vi "testDoubleArrayToStringWithBrackets.vi"(8 "error in (no error)":errorcluster) -> (0 "error out":errorcluster)   [LabVIEW 2018]
uses:
  <vilib>/addons/_JKI Toolkits/Caraya/classes/Assert/Assert Equal Value_Variant.vi
  <vilib>/addons/_JKI Toolkits/Caraya/classes/Test/Test.lvclass
  <vilib>/addons/_JKI Toolkits/Caraya/classes/Assert/Assert.lvclass
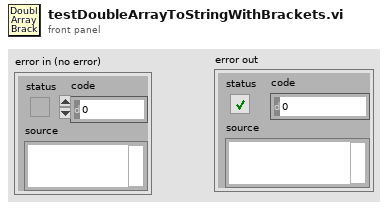
[diagram p1: front panel]
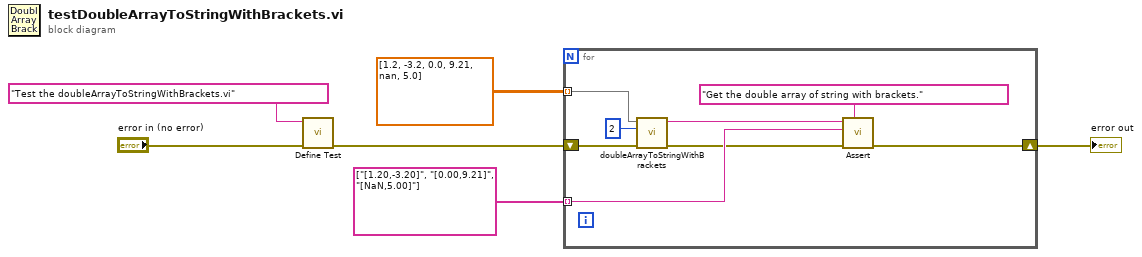
[diagram p0: block diagram]
diagram:
  n1 = call <vilib>:"Define Test.vi"("error in (no error)"="error in (no error)", "Label (VI Title)"="Test the doubleArrayToStringWithBrackets.vi") -> ("error out"=w1:errorcluster)  [unwired: 9 in]
  n2 = for {
    tunnel: string[] ["[1.20,-3.20]", "[0.00,9.21]", "[NaN,5.00]"] ("name") -> [w13] mode=indexing
    shift-right: [w12] -> w3
    shift-left: w1 -> [w8]
    tunnel: dbl[][] [[1.2, -3.2], [0.0, 9.21], [nan, 5.0]] ("value") -> [w11] mode=indexing
    n3 = call "doubleArrayToStringWithBrackets.vi"("error in (no error)"=w8, "presicion (0)"=u8 2, "value"=w11) -> ("error out"=w7:errorcluster, "String"=w10:string)  [unwired: 7 in]
    n4 = call-poly <vilib>:"Assert.vi"("Label"="Get the double array of string with brackets.", "error in (no error)"=w7, "Y"=w13, "X"=w10) -> ("error out"=w12:errorcluster)  [unwired: 7 in]
  }
  "error out" <- w3
